vi "Configure Frequency Sweep.vi"(4 "Stop  Frequency (1000.0 Hz)":dbl=1000.0 format="%#.6g", 6 "Start Frequency (100.0 Hz)":dbl=100.0 format="%#.6g", 7 "Enable Frequency Sweep Mode (T: Enable)":bool=TRUE, 8 "error in (no error)":errorcluster, 9 "Sweep Time (1.00 s)":dbl=1.0 format="%#.6g", 10 "Sweep Spacing (0: Linear)":u16(ring) items=["Linear", "Logarithmic"], 11 "VISA resource name":refnum<visa-resource-name>) -> (0 "error out":errorcluster, 3 "VISA resource name out":refnum<visa-resource-name>)   [LabVIEW 2012, in "Agilent 33XXX Series.lvlib"]
doc: "Configures and enables a frequency sweep. In the frequency sweep mode, the function generator steps from the start frequency to the stop frequency at a sweep rate."
uses:
  <instrlib>/Agilent 33XXX Series/Agilent 33XXX Series.lvlib
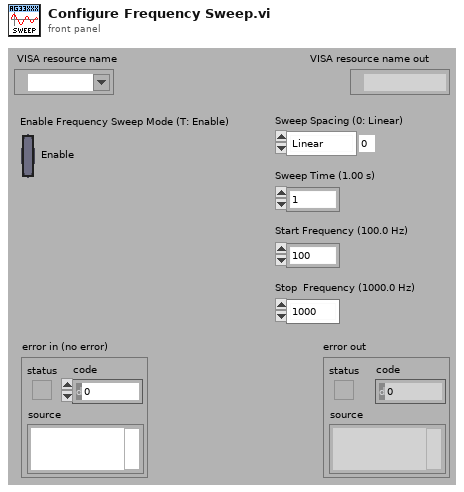
[diagram p1: front panel]
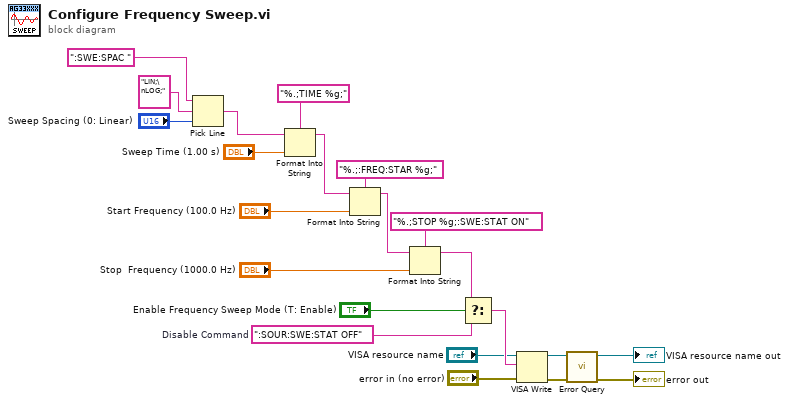
[diagram p0: block diagram]
diagram:
  w7 = ":SOUR:SWE:STAT OFF"  # Disable Command
  n1 = Pick Line(string ("")=":SWE:SPAC ", multi-line string="LIN;\nLOG;", line index="Sweep Spacing (0: Linear)") -> (output string=w9:string)
  n2 = Format Into String(format string="%.;TIME %g;", initial string=w9, "Sweep Time (1.00 s)") -> (resulting string=w17:string)  [unwired: 1 in, 1 out]
  n3 = Format Into String(format string="%.;:FREQ:STAR %g;", initial string=w17, "Start Frequency (100.0 Hz)") -> (resulting string=w14:string)  [unwired: 1 in, 1 out]
  n4 = Format Into String(format string="%.;STOP %g;:SWE:STAT ON", initial string=w14, "Stop  Frequency (1000.0 Hz)") -> (resulting string=w6:string)  [unwired: 1 in, 1 out]
  n5 = Select(t=w6, s="Enable Frequency Sweep Mode (T: Enable)", f=w7) -> (s? t:f=w8:string)
  n6 = VISA Write(VISA resource name="VISA resource name", write buffer=w8, error in (no error)="error in (no error)") -> (VISA resource name out=w22:refnum<visa-resource-name>, error out=w21:errorcluster)  [unwired: 1 out]
  n7 = call <instrlib>:"Error Query.vi"("error in (no error)"=w21, "VISA resource name"=w22) -> ("error out"=→"error out":errorcluster, "VISA resource name out"=→"VISA resource name out":refnum<visa-resource-name>)  [unwired: 6 in, 2 out]
